vi "NicmosAcquisition.vi"(3 "Acquisition":i32, 9 "error in (no error)":errorcluster caption="error out (no error)") -> (0 "DATA":T1, 6 "error out":errorcluster)   [LabVIEW 2009]
uses:
  Controls/NICMOS.DATA.ARRAY.ctl
  Controls/NICMOS.DATA.ctl
  Controls/NICMOS.COMMAND.ctl
  Controls/NICMOS.COMMANDBASIC.ctl
  Controls/NICMOS.READOUT.ctl
  Controls/NICMOS.FILTERCOMMAND.ctl
  Controls/NICMOS.FILTER.ctl
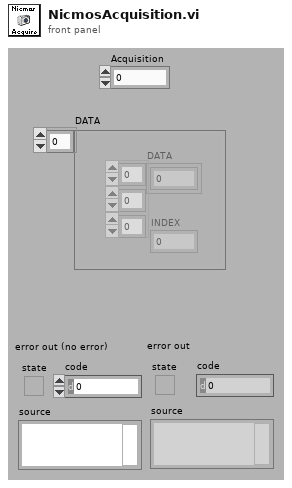
[diagram p1: front panel]
types:
  T1 = typedef "NICMOS.DATA.ARRAY.ctl" = T2[]
  T2 = typedef "NICMOS.DATA.ctl" = cluster{"DATA":i32[][][], "INDEX":i32}
  T3 = typedef "NICMOS.COMMAND.ctl" = cluster{"Command":T4, "READOUT":T5, "FILTERCOMMAND":T6, "ACQUISITION":i32, "Done":refnum<k4>}
  T4 = typedef "NICMOS.COMMANDBASIC.ctl" = enum16{"WRITE BANKS", "SET FILTER", "HOME FILTER", "QUERY TEMP", "CONFIGURE", "START", "ACQUISITION", "STOP", "QUIT"}
  T5 = typedef "NICMOS.READOUT.ctl" = cluster{"Readout":i32, "Deglitch":i32, "Framerate":dbl[unit], "Bank":i32}
  T6 = typedef "NICMOS.FILTERCOMMAND.ctl" = cluster{"FILTER":T7, "INIT":bool}
  T7 = typedef "NICMOS.FILTER.ctl" = string
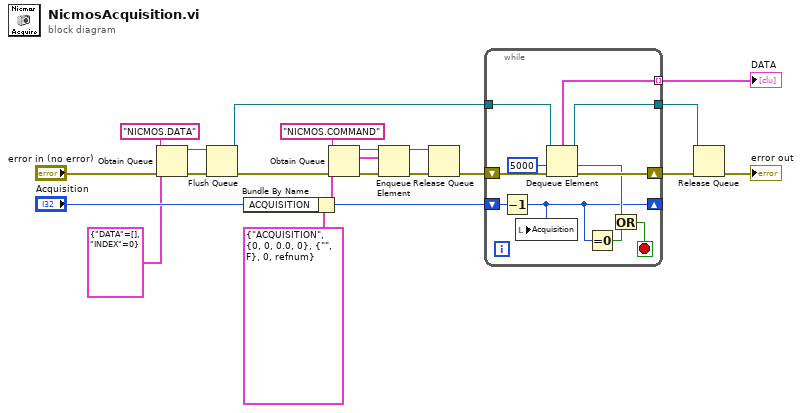
[diagram p0: block diagram]
diagram:
  n1 = Obtain Queue(name (unnamed)="NICMOS.DATA" ("nom (aucun)"), element data type=T2 {"DATA"=[], "INDEX"=0} ("DATA"), error in (no error)="error in (no error)") -> (queue out=w2:refnum<queue>, error out=w4:errorcluster)  [unwired: 2 in, 1 out]
  n2 = Flush Queue(queue=w2, error in (no error)=w4) -> (queue out=w1:refnum<queue>, error out=w3:errorcluster)  [unwired: 1 out]
  n3 = Bundle By Name(cluster=T3 {"Command"=enum."ACQUISITION", "READOUT"={"Readout"=0, "Deglitch"=0, "Framerate"=0.0, "Bank"=0}, "FILTERCOMMAND"={"FILTER"="", "INIT"=FALSE}, "ACQUISITION"=0, "Done"=refnum} ("COMMAND"), "ACQUISITION"="Acquisition") -> (w17:T3)
  n4 = Obtain Queue(name (unnamed)="NICMOS.COMMAND" ("nom (aucun)"), element data type=w17, error in (no error)=w3) -> (queue out=w19:refnum<queue>, error out=w18:errorcluster)  [unwired: 2 in, 1 out]
  n5 = Enqueue Element(queue=w19, element=w17, error in (no error)=w18) -> (queue out=w16:refnum<queue>, error out=w15:errorcluster)  [unwired: 1 in, 1 out]
  n6 = Release Queue(queue=w16, error in (no error)=w15) -> (error out=w11:errorcluster)  [unwired: 1 in, 2 out]
  n7 = while {
    tunnel: w1 -> [w25]
    shift-right: [w29] -> w9
    shift-left: w11 -> [w31]
    shift-right: [w21] -> _
    shift-left: "Acquisition" -> [w28]
    tunnel: [w24] -> w7
    tunnel: [w23] -> w5 mode=indexing
    stop <- w22 stop-if-true
    n8 = Decrement(x=w28) -> (x-1=w21:i32)
    n9 = local write "Acquisition"(w21) -> ()
    n10 = Dequeue Element(queue=w25, timeout in ms (-1)=5000 ("timeout en ms (-1)"), error in (no error)=w31) -> (queue out=w24:refnum<queue>, element=w23:T2, timed out?=w26:bool, error out=w29:errorcluster)
    n11 = Equal To 0?(x=w21) -> (x = 0?=w27:bool)
    n12 = Or(x=w26, y=w27) -> (x .or. y?=w22:bool)
  }
  "DATA" <- w5
  n13 = Release Queue(queue=w7, error in (no error)=w9) -> (error out=→"error out":errorcluster)  [unwired: 1 in, 2 out]
